vi "Lab2.vi"() -> ()   [LabVIEW 2015, in "Task 2 Labview.lvrbt"]
uses:
  Task 2 Labview.lvrbt
  <vilib>/NXT/Block Support/NXT_InputPort.ctl
  <vilib>/NXT/Block Support/NXT_OutputPort.ctl
  <vilib>/NXT/Subs/MotorOutput.ctl
  <vilib>/NXT/Dual Mode Library/Display/drawText.vi
  <vilib>/NXT/NXTIO Xnodes/NXTIONodeSubVIs/NXTMoveMotors.vi
  <vilib>/NXT/Dual Mode Library/Waits/Wait_Num.vi
  <vilib>/NXT/Dual Mode Library/Sensors/EV3_Color_Reflect.vi
  <vilib>/NXT/NXTIO Xnodes/NXTIONodeSubVIs/LEGOStopAllMotors.vi
  <vilib>/NXT/Dual Mode Library/Waits/Wait_Bump.vi
  <vilib>/NXT/Dual Mode Library/Display/clearDisplay.vi
  <vilib>/NXT/Dual Mode Library/Waits/Wait_Num(msec).vi
  <vilib>/NXT/Dual Mode Library/Sensors/Touch_Pressed.vi
  <vilib>/NXT/Dual Mode Library/Sensors/EV3_Touch_Reset.vi
  <vilib>/NXT/Dual Mode Library/Sensors/EV3_Ultrasonic_CM.vi
  <vilib>/NXT/Dual Mode Library/Motors/MotorBrake.vi
  <vilib>/NXT/Dual Mode Library/Motors/MotorOn.vi
  <vilib>/NXT/Dual Mode Library/Waits/Wait_LetGo.vi
  <vilib>/NXT/NXTIO Xnodes/AddressXNode/NXTIOAddress.xnode
  <vilib>/NXT/NXTIO Xnodes/NXTIOXNode/NXTIO.xnode
  <vilib>/NXT/Subs/LVHSConnector.ctl
  <vilib>/NXT/LegoClasses/BrickReference/BrickReference.lvclass
panel:
  out "Scaled Value 2":sgl
  out "Scaled Value":sgl
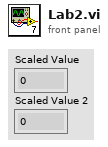
[diagram p1: front panel]
types:
  T1 = typedef "NXT_InputPort.ctl" = u32
  T2 = typedef "NXT_OutputPort.ctl" = u8
  T3 = typedef "LVHSConnector.ctl" = refnum<class "BrickReference.lvclass">
  T4 = typedef "MotorOutput.ctl" = u8
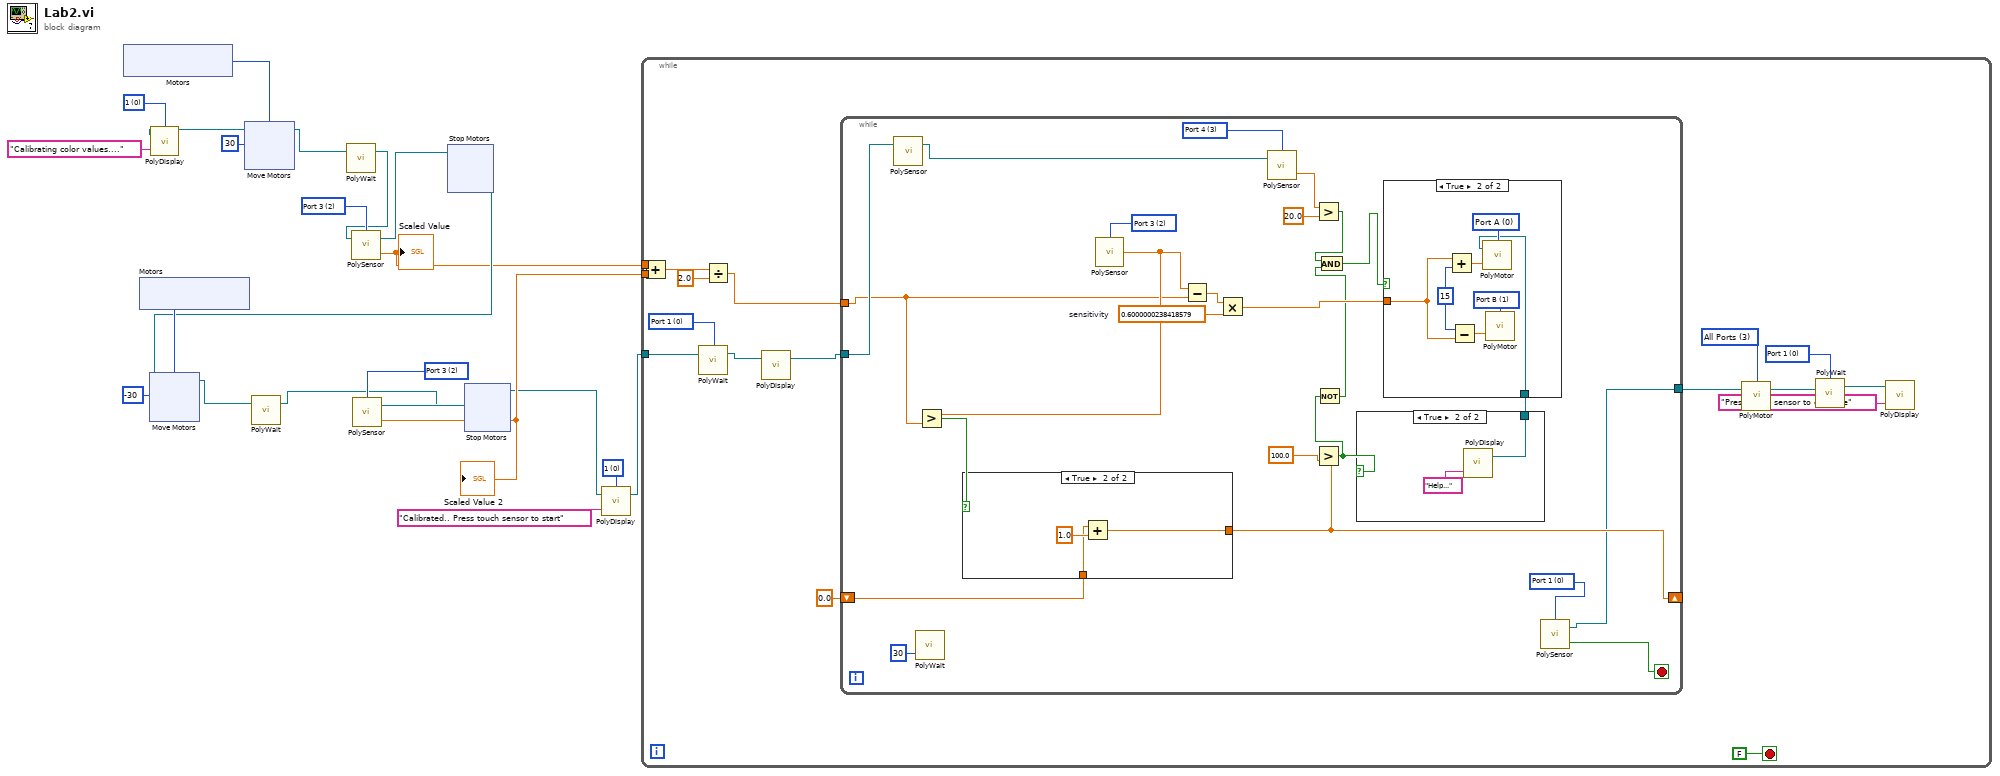
[diagram p0: block diagram]
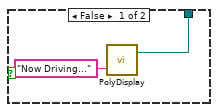
[diagram p2: hidden frame]
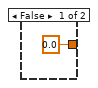
[diagram p3: hidden frame]
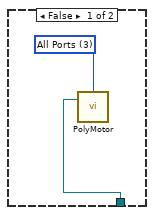
[diagram p4: hidden frame]
diagram:
  w5 = i16 0 items=["1", "2", "3", "4", "5", "6", "7", "8", "9", "10", "11", "12"] ("Line")
  w14 = T1 2 items=["Port 1", "Port 2", "Port 3", "Port 4"] ("Port (Port 1)")
  w15 = T1 2 items=["Port 1", "Port 2", "Port 3", "Port 4"] ("Port (Port 1)")
  w22 = i16 0 items=["1", "2", "3", "4", "5", "6", "7", "8", "9", "10", "11", "12"] ("Line")
  n1 = xnode "Motors"() -> ("Motor"=w20:T2)
  n2 = xnode "Motors"() -> ("Motor"=w17:T2)
  n3 = call-poly <vilib>:"PolyDisplay.vi"("Text"="Calibrating color values....", "Line"=w22) -> ("NXT/EV3"=w7:T3)  [unwired: 2 in]
  n4 = xnode "Move Motors"("Power/Speed 1"=i8 30, "Motors"=w20, "NXT/EV3"=w7) -> ("NXT/EV3"=w19:T3)
  n5 = call-poly <vilib>:"PolyWait.vi"("NXT/EV3"=w19) -> ("NXT/EV3"=w11:T3)  [unwired: 3 in]
  n6 = call-poly <vilib>:"PolySensor.vi"("NXT/EV3"=w11, "Port (Port 1)"=w15) -> ("Scaled Value"=w1:sgl, "NXT/EV3"=w12:T3)  [unwired: 1 in]
  "Scaled Value" <- w1
  n7 = xnode "Stop Motors"("NXT/EV3"=w12) -> ("NXT/EV3"=w8:T3)  [unwired: 1 in]
  n8 = xnode "Move Motors"("Power/Speed 1"=i8 -30, "Motors"=w17, "NXT/EV3"=w8) -> ("NXT/EV3"=w18:T3)
  n9 = call-poly <vilib>:"PolyWait.vi"("NXT/EV3"=w18) -> ("NXT/EV3"=w9:T3)  [unwired: 3 in]
  n10 = call-poly <vilib>:"PolySensor.vi"("NXT/EV3"=w9, "Port (Port 1)"=w14) -> ("Scaled Value"=w6:sgl, "NXT/EV3"=w10:T3)  [unwired: 1 in]
  "Scaled Value 2" <- w6
  n11 = xnode "Stop Motors"("NXT/EV3"=w10) -> ("NXT/EV3"=w3:T3)  [unwired: 1 in]
  n12 = call-poly <vilib>:"PolyDisplay.vi"("Text"="Calibrated.. Press touch sensor to start", "NXT/EV3"=w3, "Line"=w5) -> ("NXT/EV3"=w2:T3)  [unwired: 1 in]
  n13 = while {
    tunnel: w6 -> [w35]
    tunnel: w1 -> [w34]
    tunnel: w2 -> [w30]
    stop <- FALSE stop-if-true
    w25 = T1 0 items=["Port 1", "Port 2", "Port 3", "Port 4"] ("Port (Port 1)")
    w26 = T1 0 items=["Port 1", "Port 2", "Port 3", "Port 4"] ("Port (Port 1)")
    w39 = T4 3 items=["Port A"=0, "Port B"=1, "Port C"=2, "Ports A & B"=4, "Ports A & C"=5, "Ports B & C"=6, "All Ports"=3] ("Port (All Ports)")
    n14 = Add(x=w34, y=w35) -> (x+y=w38:sgl)
    n15 = call-poly <vilib>:"PolyWait.vi"("NXT/EV3"=w30, "Port (Port 1)"=w25) -> ("NXT/EV3"=w29:T3)  [unwired: 2 in]
    n16 = Divide(x=w38, y=sgl 2.0) -> (x/y=w36:sgl)
    n17 = call-poly <vilib>:"PolyDisplay.vi"("NXT/EV3"=w29) -> ("NXT/EV3"=w28:T3)  [unwired: 3 in]
    n18 = while {
      tunnel: w36 -> [w52]
      tunnel: w28 -> [w55]
      tunnel: [w40] -> w33
      shift-right: [w47] -> _
      shift-left: 0.0 -> [w50]
      stop <- w42 stop-if-true
      w41 = T1 0 items=["Port 1", "Port 2", "Port 3", "Port 4"] ("Port (Port 1)")
      w58 = T1 3 items=["Port 1", "Port 2", "Port 3", "Port 4"] ("Port (Port 1)")
      w60 = sgl 0.6  # sensitivity
      w63 = T1 2 items=["Port 1", "Port 2", "Port 3", "Port 4"] ("Input Port (Port 3)")
      n19 = call-poly <vilib>:"PolySensor.vi"("NXT/EV3"=w55) -> ("NXT/EV3"=w54:T3)  [unwired: 3 in]
      n20 = call-poly <vilib>:"PolyWait.vi"("Time (100 msec)"=u32 30 ("Time (1 sec)")) -> ()  [unwired: 3 in, 1 out]
      n21 = call-poly <vilib>:"PolySensor.vi"("Port (Port 1)"=w63) -> ("Scaled Value"=w53:sgl)  [unwired: 1 in, 2 out]
      n22 = Greater?(x=w53, y=w52) -> (0:w51:bool)
      n23 = case shown="True" w51 {
        tunnel: [0.0 w70] -> w47
        tunnel: w50 -> [_ w69]
        frame False {
        }
        frame True {
          n24 = Add(x=w69, y=1.0) -> (x+y=w70:dbl)
        }
      }
      n25 = Subtract(x=w53, y=w52) -> (x-y=w61:sgl)
      n26 = Multiply(x=w61, y=w60) -> (x*y=w59:sgl)
      n27 = call-poly <vilib>:"PolySensor.vi"("NXT/EV3"=w54, "Port (Port 1)"=w58) -> ("Centimeters"=w57:sgl)  [unwired: 1 in, 1 out]
      n28 = Greater?(x=w57, y=sgl 20.0) -> (0:w45:bool)
      n29 = Greater?(x=w47, y=100.0) -> (0:w46:bool)
      n30 = Not(x=w46) -> (.not. x?=w44:bool)
      n31 = And(x=w45, y=w44) -> (x .and. y?=w43:bool)
      n32 = case shown="True" w46 {
        tunnel: [w64 w66] -> w48
        frame False {
          n33 = call-poly <vilib>:"PolyDisplay.vi"("Text"="Now Driving...") -> ("NXT/EV3"=w64:T3)  [unwired: 3 in]
        }
        frame True {
          n34 = call-poly <vilib>:"PolyDisplay.vi"("Text"="Help...") -> ("NXT/EV3"=w66:T3)  [unwired: 3 in]
        }
      }
      n35 = case shown="True" w43 {
        tunnel: w59 -> [_ w75]
        tunnel: w48 -> [w72 w74]
        frame False {
          w73 = T4 3 items=["Port A"=0, "Port B"=1, "Port C"=2, "Ports A & B"=4, "Ports A & C"=5, "Ports B & C"=6, "All Ports"=3] ("Port (All Ports)")
          n36 = call-poly <vilib>:"PolyMotor.vi"("NXT/EV3"=w72, "Port (All Ports)"=w73) -> ()  [unwired: 3 out]
        }
        frame True {
          w76 = T4 1 items=["Port A"=0, "Port B"=1, "Port C"=2, "Ports A & B"=4, "Ports A & C"=5, "Ports B & C"=6, "All Ports"=3] ("Output Port (All Ports)")
          w77 = T4 0 items=["Port A"=0, "Port B"=1, "Port C"=2, "Ports A & B"=4, "Ports A & C"=5, "Ports B & C"=6, "All Ports"=3] ("Output Port (All Ports)")
          w79 = 15 ("y")
          n37 = Add(x=w75, y=w79) -> (x+y=w80:sgl)
          n38 = Subtract(x=w79, y=w75) -> (x-y=w78:sgl)
          n39 = call-poly <vilib>:"PolyMotor.vi"("Power (75)"=w80, "NXT/EV3"=w74, "Output Port (All Ports)"=w77) -> ()  [unwired: 2 out]
          n40 = call-poly <vilib>:"PolyMotor.vi"("Power (75)"=w78, "Output Port (All Ports)"=w76) -> ()  [unwired: 1 in, 2 out]
        }
      }
      n41 = call-poly <vilib>:"PolySensor.vi"("Port (Port 1)"=w41) -> ("Yes / No"=w42:bool, "NXT/EV3"=w40:T3)  [unwired: 2 in]
    }
    n42 = call-poly <vilib>:"PolyMotor.vi"("NXT/EV3"=w33, "Port (All Ports)"=w39) -> ("NXT/EV3"=w27:T3)  [unwired: 2 out]
    n43 = call-poly <vilib>:"PolyWait.vi"("NXT/EV3"=w27, "Port (Port 1)"=w26) -> ("NXTEV3"=w24:T3)  [unwired: 2 in]
    n44 = call-poly <vilib>:"PolyDisplay.vi"("Text"="Press touch sensor to continue", "NXT/EV3"=w24) -> ()  [unwired: 2 in, 1 out]
  }
